vi "Raycaster_Run.vi"   [LabVIEW 2020]
uses:
  Controls/Raycaster_PlayLoop.ctl
  Controls/Game_State.ctl
  Controls/Player_LocationInfo.ctl
  Controls/Player_LocationInfoAxis.ctl
  Controls/Map_Position.ctl
  Controls/Map_Objects.ctl
  Controls/Map_Object.ctl
  Controls/Raycaster_DrawState.ctl
  Globals/FGV_TileVisibleEnum.ctl
  Raycaster_SetupDDA.vi
  Raycaster_RunDDA.vi
  Raycaster_DrawColumnSimple.vi
  Raycaster_CalcWallDistance.vi
  Raycaster_CalcWallHeight.vi
  Raycaster_GetSubBufferAddress.vi
  Raycaster_WriteFramebuffer.vi
  Globals/WIDTH.vi
  Math_Multiply_FXP.vi
  Math_Add_FXP.vi
  Math_Reciprocal.vi
  Math_Subtract_FXP.vi
  Globals/MAP_DIM.vi
  Map_ReadValue.vi
  Math_Divide_FXP.vi
  Globals/HEIGHT_DIV_2.vi
  Map_GetMaps.vi
  <vilib>/Utility/file.llb/Application Directory.vi
  <vilib>/eio/EIONode/EIONode.xnode
  <vilib>/rvi/DataTransferAndStorage/Container/XNode/niFpgaContainer.xnode
  <vilib>/rvi/Memory/Memory_Emulation/nirvimemoryEmulation.vi
  <vilib>/rvi/Memory/Memory_Emulation/nirvimemoryFastEmulation.vi
  <vilib>/rvi/eio/common/nirviEmuTemplateMethod_errors.vi
types:
  T1 = typedef "Map_Object.ctl" = cluster{"Distance":fxp<+/-,32,16>, "ID":u8, "Position":T2, "Visible":bool}
  T2 = typedef "Map_Position.ctl" = cluster{"X":fxp<+/-,32,16>, "Y":fxp<+/-,32,16>}
  T3 = typedef "Map_Objects.ctl" = cluster{"Objects":T1[], "Num Objects":i16, "Visible Objects":i16}
  T4 = typedef "Game_State.ctl" = cluster{"Map":u8, "Map Address":u32, "Location Info":T5, "Elevator":T2}
  T5 = typedef "Player_LocationInfo.ctl" = cluster{"X":T6, "Y":T6}
  T6 = typedef "Player_LocationInfoAxis.ctl" = cluster{"Position":fxp<+/-,32,16>, "Direction":fxp<+/-,32,16>, "Plane":fxp<+/-,32,16>}
  T7 = typedef "Raycaster_PlayLoop.ctl" = enum16{"Init", "Read Inputs", "Move Doors", "Move Walls", "Draw Walls", "Init Ray Caster", "Draw Scaled", "Draw Fizzle", "Update Screen"}
  T8 = typedef "Raycaster_DrawState.ctl" = cluster{"Buffer 0":u8[], "Buffer 1":u8[], "Buffer 2":u8[], "Buffer 3":u8[], "Wall Height 0":i16[], "Wall Height 1":i16[], "Wall Height 2":i16[], "Wall Height 3":i16[]}
  T9 = typedef "FGV_TileVisibleEnum.ctl" = enum16{"Reset", "Set Value", "Read Value"}
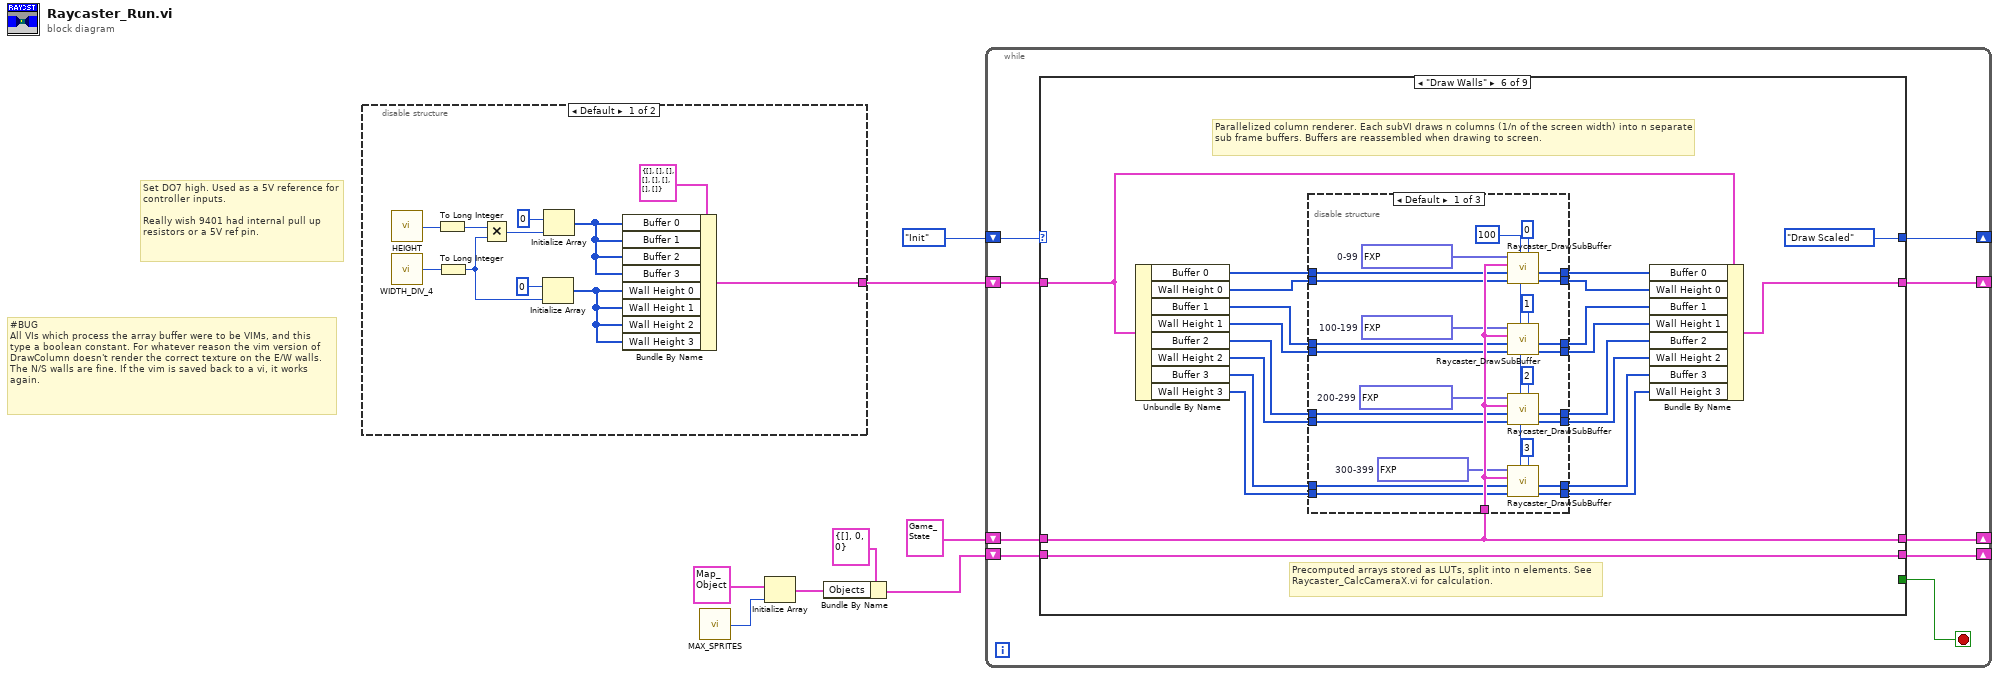
[diagram p0: block diagram]
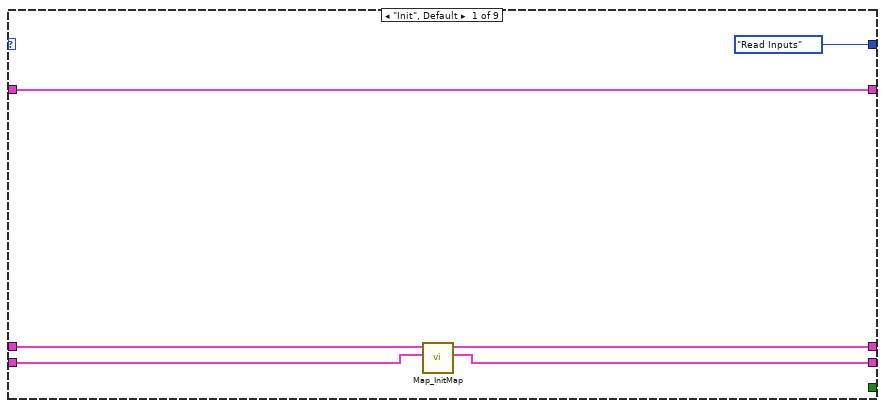
[diagram p2: hidden frame]
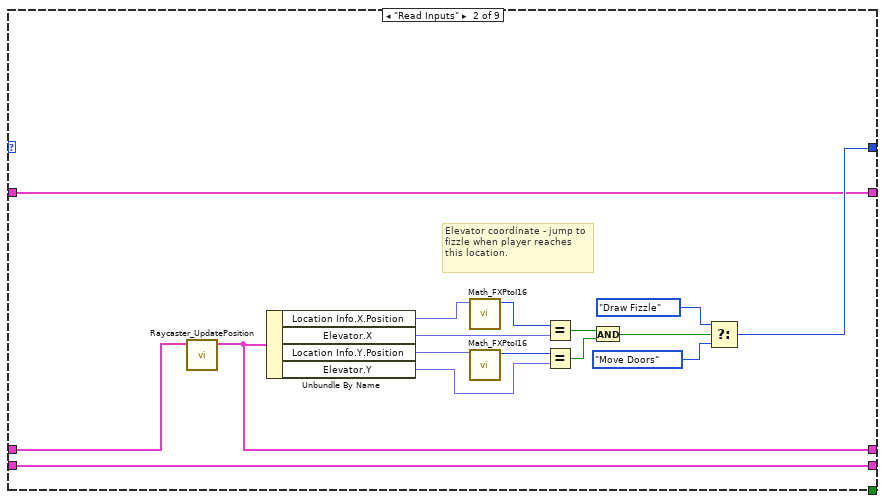
[diagram p3: hidden frame]
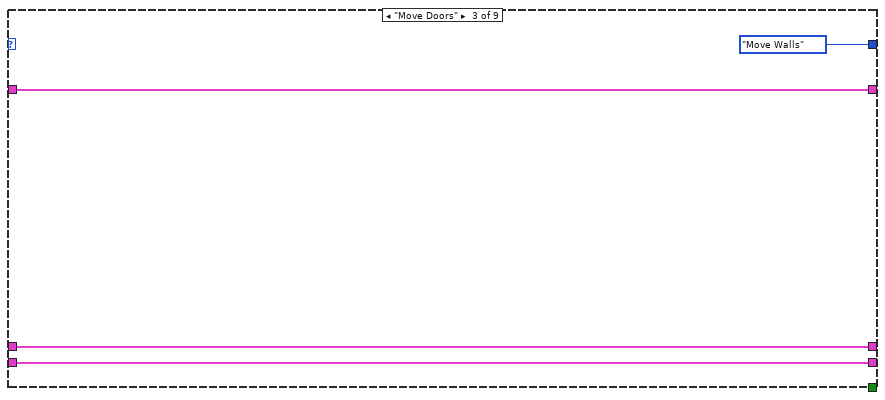
[diagram p4: hidden frame]
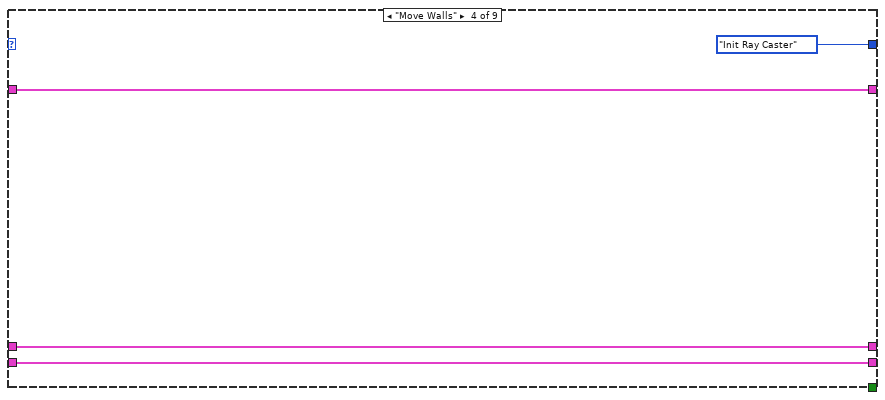
[diagram p5: hidden frame]
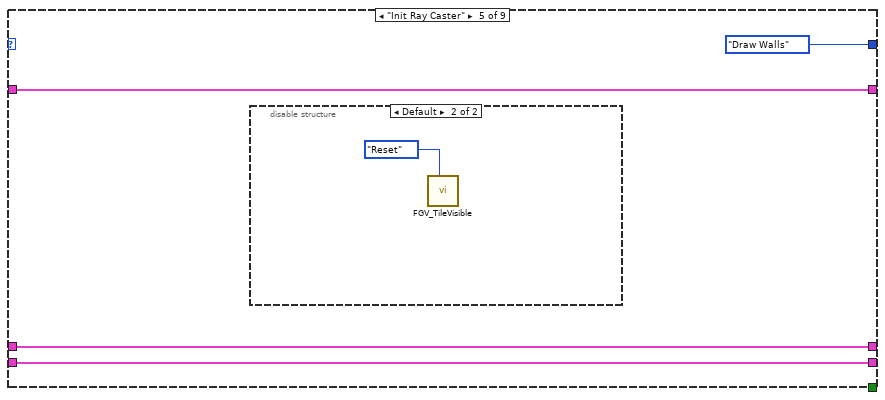
[diagram p6: hidden frame]
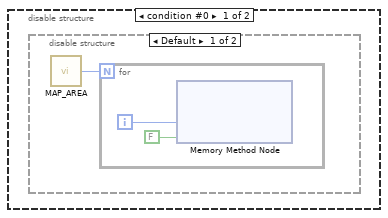
[diagram p7: hidden frame]
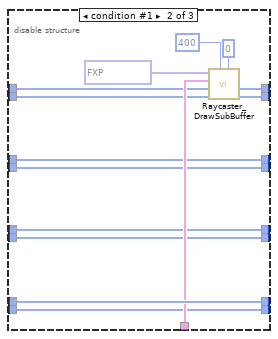
[diagram p9: hidden frame]
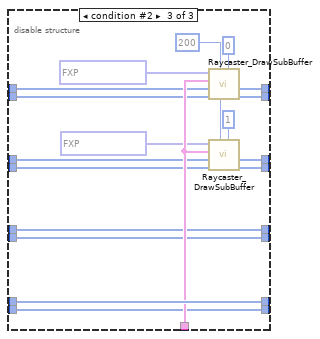
[diagram p10: hidden frame]
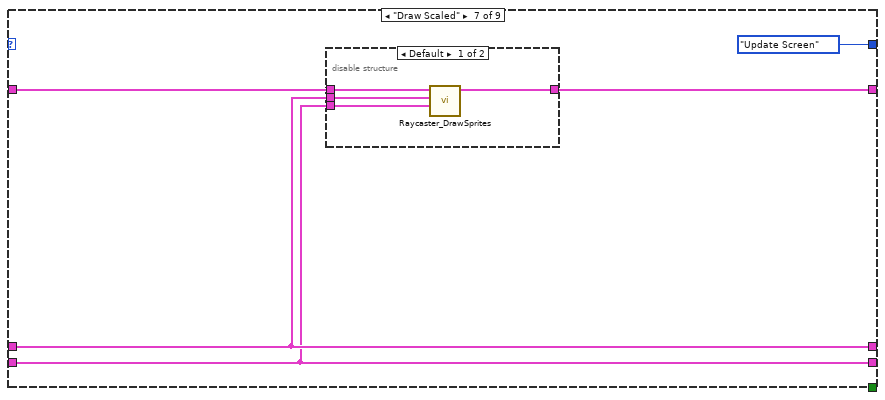
[diagram p11: hidden frame]
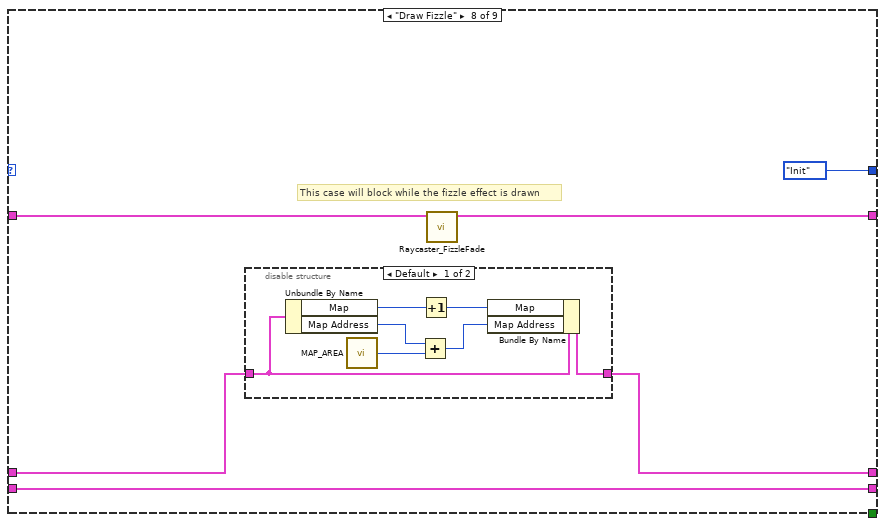
[diagram p13: hidden frame]
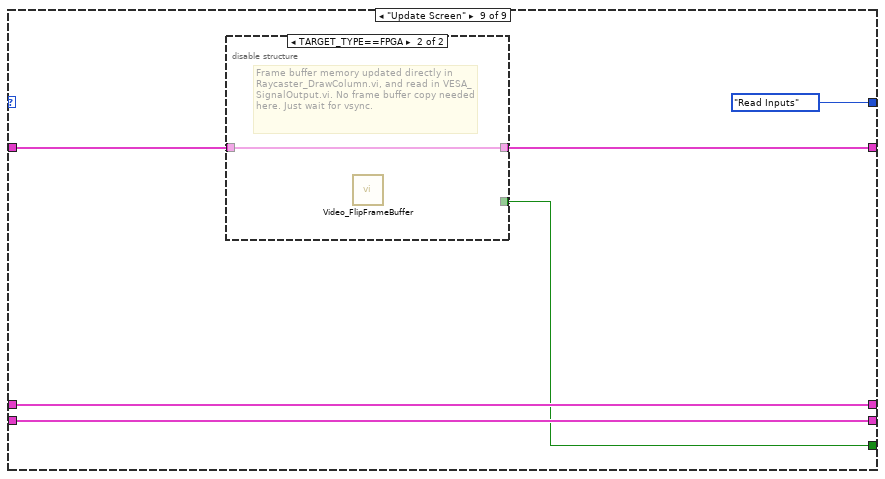
[diagram p15: hidden frame]
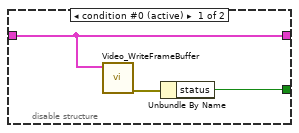
[diagram p16: hidden frame]
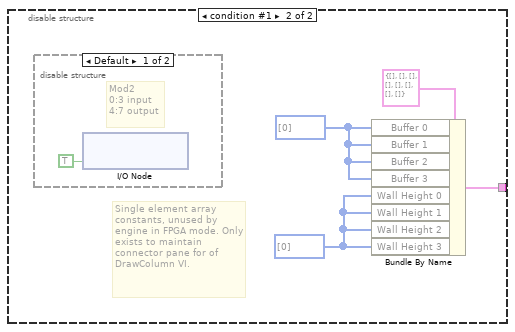
[diagram p17: hidden frame]
diagram:
  # "Set DO7 high. Used as a 5V reference for controller inputs.\n\nReally wish 9401 had internal pull up resistors or a 5V ref pin."
  # "#BUG\nAll VIs which process the array buffer were to be VIMs, and this type a boolean constant. For whatever reason the vim version of DrawColumn doesn't render the correct texture on the E/W walls. The N/S walls are fine. If the vim is saved back to a vi, it works again."
  n1 = disable-structure "Conditional Disable Structure" shown="Default" {
    disable-tunnel: [w15 w21] -> w2
    frame condition #0 (active) {
      n2 = call "HEIGHT.vi"() -> ("HEIGHT"=w19:i16)
      n3 = call "WIDTH_DIV_4.vi"() -> ("WIDTH_DIV_4"=w12:i16)
      n4 = To Long Integer(number=w19) -> (32bit integer=w18:i32)
      n5 = To Long Integer(number=w12) -> (32bit integer=w9:i32)
      n6 = Multiply(x=w18, y=w9) -> (x*y=w14:i32)
      n7 = Initialize Array(i16 0, w9) -> (w10:i16[])
      n8 = Initialize Array(u8 0, w14) -> (w13:u8[])
      n9 = Bundle By Name(cluster=T8 {"Buffer 0"=[], "Buffer 1"=[], "Buffer 2"=[], "Buffer 3"=[], "Wall Height 0"=[], "Wall Height 1"=[], "Wall Height 2"=[], "Wall Height 3"=[]} ("Frame buffers"), "Buffer 0"=w13, "Buffer 1"=w13, "Buffer 2"=w13, "Buffer 3"=w13, "Wall Height 0"=w10, "Wall Height 1"=w10, "Wall Height 2"=w10, "Wall Height 3"=w10) -> (w15:T8)
    }
    frame condition #1 {
      w20 = i16[] [0]
      w22 = u8[] [0]
      # "Single element array constants, unused by engine in FPGA mode. Only exists to maintain connector pane for of DrawColumn VI."
      n10 = disable-structure "Conditional Disable Structure" shown="Default" {
        frame condition #0 (active) {
          # "Mod2\n0:3 input\n4:7 output"
          n11 = xnode ("I/O Node")("Mod2/DIO7"=TRUE) -> ()  [unwired: 1 in, 1 out]
        }
        frame condition #1 {
        }
      }
      n12 = Bundle By Name(cluster=T8 {"Buffer 0"=[], "Buffer 1"=[], "Buffer 2"=[], "Buffer 3"=[], "Wall Height 0"=[], "Wall Height 1"=[], "Wall Height 2"=[], "Wall Height 3"=[]} ("Frame buffers"), "Buffer 0"=w22, "Buffer 1"=w22, "Buffer 2"=w22, "Buffer 3"=w22, "Wall Height 0"=w20, "Wall Height 1"=w20, "Wall Height 2"=w20, "Wall Height 3"=w20) -> (w21:T8)
    }
  }
  n13 = call "MAX_SPRITES.vi"() -> ("MAX_SPRITES"=w1:u8)
  n14 = Initialize Array(T1 {"Distance"=0.0, "ID"=0, "Position"={"X"=0.0, "Y"=0.0}, "Visible"=FALSE} ("Object"), w1) -> (w5:T1[])
  n15 = Bundle By Name(cluster=T3 {"Objects"=[], "Num Objects"=0, "Visible Objects"=0} ("Map Objects"), "Objects"=w5) -> (w3:T3)
  n16 = while {
    shift-right: [w29] -> _
    shift-left: T4 {"Map"=0, "Map Address"=0, "Location Info"={"X"={"Position"=0.0, "Direction"=0.0, "Plane"=0.0}, "Y"={"Position"=0.0, "Direction"=0.0, "Plane"=0.0}}, "Elevator"={"X"=0.0, "Y"=0.0}} ("Game State") -> [w30]
    shift-right: [w31] -> _
    shift-left: Raycaster_PlayLoop."Init" -> [w32]
    shift-right: [w26] -> _
    shift-left: w2 -> [w33]
    shift-right: [w27] -> _
    shift-left: w3 -> [w28]
    stop <- w25 stop-if-true
    n17 = case shown="\"Draw Walls\"" w32 {
      tunnel: w33 -> [w34 w51 w56 w60 w64 w89 w154 w162 w179]
      tunnel: [w37 w54 w58 w62 w66 w91 w153 w165 w180] -> w29
      tunnel: [Raycaster_PlayLoop."Read Inputs" w53 Raycaster_PlayLoop."Move Walls" Raycaster_PlayLoop."Init Ray Caster" Raycaster_PlayLoop."Draw Walls" Raycaster_PlayLoop."Draw Scaled" Raycaster_PlayLoop."Update Screen" Raycaster_PlayLoop."Init" Raycaster_PlayLoop."Read Inputs"] -> w31
      tunnel: w30 -> [w38 w55 w58 w62 w66 w91 w153 w164 w180]
      tunnel: w28 -> [w36 w52 w57 w61 w65 w90 w152 w163 w177]
      tunnel: [w35 w52 w57 w61 w65 w90 w152 w163 w177] -> w27
      tunnel: [w34 w51 w56 w60 w64 w88 w151 w161 w176] -> w26
      tunnel: [_ _ _ _ _ _ _ _ w175] -> w25
      frame "Init", Default {
        n18 = call "Map_InitMap.vi"("Map Objects In"=w36, "Game State In"=w38) -> ("Map Objects Out"=w35:T3, "Game State Out"=w37:T4)  [unwired: 8 in]
      }
      frame "Read Inputs" {
        # "Elevator coordinate - jump to fizzle when player reaches this location."
        n19 = call "Raycaster_UpdatePosition.vi"("Game State In"=w55) -> ("Game State Out"=w54:T4)  [unwired: 10 in]
        n20 = Unbundle By Name(w54) -> ("Location Info.X.Position"=w50:fxp<+/-,32,16>, "Elevator.X"=w41:fxp<+/-,32,16>, "Location Info.Y.Position"=w42:fxp<+/-,32,16>, "Elevator.Y"=w40:fxp<+/-,32,16>)
        n21 = call "Math_FXPtoI16.vi"("FXP"=w50) -> ("I16"=w49:i16)  [unwired: 10 in]
        n22 = call "Math_FXPtoI16.vi"("FXP"=w42) -> ("I16"=w48:i16)  [unwired: 10 in]
        n23 = Equal?(x=w49, y=w41) -> (x = y?=w47:bool)
        n24 = Equal?(x=w48, y=w40) -> (x = y?=w46:bool)
        n25 = And(x=w47, y=w46) -> (x .and. y?=w45:bool)
        n26 = Select(t=Raycaster_PlayLoop."Draw Fizzle", s=w45, f=Raycaster_PlayLoop."Move Doors") -> (s? t:f=w53:T7)
      }
      frame "Move Doors" {
      }
      frame "Move Walls" {
      }
      frame "Init Ray Caster" {
        n27 = disable-structure "Conditional Disable Structure" shown="Default" {
          frame condition #0 {
            n28 = disable-structure shown="Default" {
              frame condition #0 (active) {
                n29 = call "MAP_AREA.vi"() -> ("MAP_DIM"=w68:i16)
                n30 = for {
                  N: w68 -> [_]
                  i -> [w69]
                  n31 = xnode ("Memory Method Node")("Address"=w69, "Data"=FALSE) -> ()  [unwired: 1 in, 1 out]
                }
              }
              frame condition #1 {
              }
            }
          }
          frame condition #1 (active) {
            n32 = call "FGV_TileVisible.vi"("Tile Visible FGV"=FGV_TileVisibleEnum."Reset") -> ()  [unwired: 10 in, 1 out]
          }
        }
      }
      frame "Draw Walls" {
        # "Parallelized column renderer. Each subVI draws n columns (1/n of the screen width) into n separate sub frame buffers. Buffers are reassembled when drawing to screen."
        # "Precomputed arrays stored as LUTs, split into n elements. See Raycaster_CalcCameraX.vi for calculation."
        n33 = Unbundle By Name(w89) -> ("Buffer 0"=w87:u8[], "Wall Height 0"=w73:i16[], "Buffer 1"=w86:u8[], "Wall Height 1"=w75:i16[], "Buffer 2"=w83:u8[], "Wall Height 2"=w77:i16[], "Buffer 3"=w82:u8[], "Wall Height 3"=w79:i16[])
        n34 = disable-structure "Conditional Disable Structure" shown="Default" {
          disable-tunnel: w91 -> [w118 w130 w148]
          disable-tunnel: w87 -> [w117 w122 w144]
          disable-tunnel: w86 -> [w116 w128 w138]
          disable-tunnel: w83 -> [w115 w129 w147]
          disable-tunnel: w82 -> [w114 w131 w149]
          disable-tunnel: [w113 w121 w142] -> w85
          disable-tunnel: [w112 w128 w137] -> w84
          disable-tunnel: [w111 w129 w147] -> w81
          disable-tunnel: [w110 w131 w149] -> w80
          disable-tunnel: w79 -> [w104 w124 w133]
          disable-tunnel: [w103 w124 w133] -> w78
          disable-tunnel: w77 -> [w100 w125 w134]
          disable-tunnel: [w99 w125 w134] -> w76
          disable-tunnel: w75 -> [w97 w126 w135]
          disable-tunnel: [w96 w126 w136] -> w74
          disable-tunnel: w73 -> [w94 w120 w141]
          disable-tunnel: [w93 w119 w140] -> w72
          frame condition #0 (active) {
            w107 = i16 100 ("Column Offset")
            w105 = fxp<+/-,32,16>[] [0.5, 0.5049896240234375, 0.5099945068359375, 0.5149993896484375, 0.519989013671875, 0.524993896484375, 0.529998779296875, 0.5349884033203125, 0.5399932861328125, 0.5449981689453125, 0.54998779296875, 0.55499267578125, 0.55999755859375, 0.5649871826171875, 0.5699920654296875, 0.5749969482421875, 0.579986572265625, 0.584991455078125, 0.589996337890625, 0.5949859619140625, 0.5999908447265625, 0.6049957275390625, 0.6099853515625, 0.614990234375, 0.6199951171875, 0.625, 0.6299896240234375, 0.6349945068359375, 0.6399993896484375, 0.644989013671875, 0.649993896484375, 0.654998779296875, 0.6599884033203125, 0.6649932861328125, 0.6699981689453125, 0.67498779296875, 0.67999267578125, 0.68499755859375, 0.6899871826171875, 0.6949920654296875, 0.6999969482421875, 0.704986572265625, 0.709991455078125, 0.714996337890625, 0.7199859619140625, 0.7249908447265625, 0.7299957275390625, 0.7349853515625, 0.739990234375, 0.7449951171875, 0.75, 0.7549896240234375, 0.7599945068359375, 0.7649993896484375, 0.769989013671875, 0.774993896484375, 0.779998779296875, 0.7849884033203125, 0.7899932861328125, 0.7949981689453125, 0.79998779296875, 0.80499267578125, 0.80999755859375, 0.8149871826171875, 0.8199920654296875, 0.8249969482421875, 0.829986572265625, 0.834991455078125, 0.839996337890625, 0.8449859619140625, 0.8499908447265625, 0.8549957275390625, 0.8599853515625, 0.864990234375, 0.8699951171875, 0.875, 0.8799896240234375, 0.8849945068359375, 0.8899993896484375, 0.894989013671875, 0.899993896484375, 0.904998779296875, 0.9099884033203125, 0.9149932861328125, 0.9199981689453125, 0.92498779296875, 0.92999267578125, 0.93499755859375, 0.9399871826171875, 0.9449920654296875, 0.9499969482421875, 0.954986572265625, 0.959991455078125, 0.964996337890625, 0.9699859619140625, 0.9749908447265625, 0.9799957275390625, 0.9849853515625, 0.989990234375, 0.9949951171875]  # 300-399
            w106 = fxp<+/-,32,16>[] [0.0, 0.0049896240234375, 0.0099945068359375, 0.0149993896484375, 0.019989013671875, 0.024993896484375, 0.029998779296875, 0.0349884033203125, 0.0399932861328125, 0.0449981689453125, 0.04998779296875, 0.05499267578125, 0.05999755859375, 0.0649871826171875, 0.0699920654296875, 0.0749969482421875, 0.079986572265625, 0.084991455078125, 0.089996337890625, 0.0949859619140625, 0.0999908447265625, 0.1049957275390625, 0.1099853515625, 0.114990234375, 0.1199951171875, 0.125, 0.1299896240234375, 0.1349945068359375, 0.1399993896484375, 0.144989013671875, 0.149993896484375, 0.154998779296875, 0.1599884033203125, 0.1649932861328125, 0.1699981689453125, 0.17498779296875, 0.17999267578125, 0.18499755859375, 0.1899871826171875, 0.1949920654296875, 0.1999969482421875, 0.204986572265625, 0.209991455078125, 0.214996337890625, 0.2199859619140625, 0.2249908447265625, 0.2299957275390625, 0.2349853515625, 0.239990234375, 0.2449951171875, 0.25, 0.2549896240234375, 0.2599945068359375, 0.2649993896484375, 0.269989013671875, 0.274993896484375, 0.279998779296875, 0.2849884033203125, 0.2899932861328125, 0.2949981689453125, 0.29998779296875, 0.30499267578125, 0.30999755859375, 0.3149871826171875, 0.3199920654296875, 0.3249969482421875, 0.329986572265625, 0.334991455078125, 0.339996337890625, 0.3449859619140625, 0.3499908447265625, 0.3549957275390625, 0.3599853515625, 0.364990234375, 0.3699951171875, 0.375, 0.3799896240234375, 0.3849945068359375, 0.3899993896484375, 0.394989013671875, 0.399993896484375, 0.404998779296875, 0.4099884033203125, 0.4149932861328125, 0.4199981689453125, 0.42498779296875, 0.42999267578125, 0.43499755859375, 0.4399871826171875, 0.4449920654296875, 0.4499969482421875, 0.454986572265625, 0.459991455078125, 0.464996337890625, 0.4699859619140625, 0.4749908447265625, 0.4799957275390625, 0.4849853515625, 0.489990234375, 0.4949951171875]  # 200-299
            w108 = fxp<+/-,32,16>[] [-0.5, -0.4950103759765625, -0.4900054931640625, -0.4850006103515625, -0.480010986328125, -0.475006103515625, -0.470001220703125, -0.4650115966796875, -0.4600067138671875, -0.4550018310546875, -0.45001220703125, -0.44500732421875, -0.44000244140625, -0.4350128173828125, -0.4300079345703125, -0.4250030517578125, -0.420013427734375, -0.415008544921875, -0.410003662109375, -0.4050140380859375, -0.4000091552734375, -0.3950042724609375, -0.3900146484375, -0.385009765625, -0.3800048828125, -0.375, -0.3700103759765625, -0.3650054931640625, -0.3600006103515625, -0.355010986328125, -0.350006103515625, -0.345001220703125, -0.3400115966796875, -0.3350067138671875, -0.3300018310546875, -0.32501220703125, -0.32000732421875, -0.31500244140625, -0.3100128173828125, -0.3050079345703125, -0.3000030517578125, -0.295013427734375, -0.290008544921875, -0.285003662109375, -0.2800140380859375, -0.2750091552734375, -0.2700042724609375, -0.2650146484375, -0.260009765625, -0.2550048828125, -0.25, -0.2450103759765625, -0.2400054931640625, -0.2350006103515625, -0.230010986328125, -0.225006103515625, -0.220001220703125, -0.2150115966796875, -0.2100067138671875, -0.2050018310546875, -0.20001220703125, -0.19500732421875, -0.19000244140625, -0.1850128173828125, -0.1800079345703125, -0.1750030517578125, -0.170013427734375, -0.165008544921875, -0.160003662109375, -0.1550140380859375, -0.1500091552734375, -0.1450042724609375, -0.1400146484375, -0.135009765625, -0.1300048828125, -0.125, -0.1200103759765625, -0.1150054931640625, -0.1100006103515625, -0.105010986328125, -0.100006103515625, -0.095001220703125, -0.0900115966796875, -0.0850067138671875, -0.0800018310546875, -0.07501220703125, -0.07000732421875, -0.06500244140625, -0.0600128173828125, -0.0550079345703125, -0.0500030517578125, -0.045013427734375, -0.040008544921875, -0.035003662109375, -0.0300140380859375, -0.0250091552734375, -0.0200042724609375, -0.0150146484375, -0.010009765625, -0.0050048828125]  # 100-199
            w109 = fxp<+/-,32,16>[] [-1.0, -0.9950103759765625, -0.9900054931640625, -0.9850006103515625, -0.980010986328125, -0.975006103515625, -0.970001220703125, -0.9650115966796875, -0.9600067138671875, -0.9550018310546875, -0.95001220703125, -0.94500732421875, -0.94000244140625, -0.9350128173828125, -0.9300079345703125, -0.9250030517578125, -0.920013427734375, -0.915008544921875, -0.910003662109375, -0.9050140380859375, -0.9000091552734375, -0.8950042724609375, -0.8900146484375, -0.885009765625, -0.8800048828125, -0.875, -0.8700103759765625, -0.8650054931640625, -0.8600006103515625, -0.855010986328125, -0.850006103515625, -0.845001220703125, -0.8400115966796875, -0.8350067138671875, -0.8300018310546875, -0.82501220703125, -0.82000732421875, -0.81500244140625, -0.8100128173828125, -0.8050079345703125, -0.8000030517578125, -0.795013427734375, -0.790008544921875, -0.785003662109375, -0.7800140380859375, -0.7750091552734375, -0.7700042724609375, -0.7650146484375, -0.760009765625, -0.7550048828125, -0.75, -0.7450103759765625, -0.7400054931640625, -0.7350006103515625, -0.730010986328125, -0.725006103515625, -0.720001220703125, -0.7150115966796875, -0.7100067138671875, -0.7050018310546875, -0.70001220703125, -0.69500732421875, -0.69000244140625, -0.6850128173828125, -0.6800079345703125, -0.6750030517578125, -0.670013427734375, -0.665008544921875, -0.660003662109375, -0.6550140380859375, -0.6500091552734375, -0.6450042724609375, -0.6400146484375, -0.635009765625, -0.6300048828125, -0.625, -0.6200103759765625, -0.6150054931640625, -0.6100006103515625, -0.605010986328125, -0.600006103515625, -0.595001220703125, -0.5900115966796875, -0.5850067138671875, -0.5800018310546875, -0.57501220703125, -0.57000732421875, -0.56500244140625, -0.5600128173828125, -0.5550079345703125, -0.5500030517578125, -0.545013427734375, -0.540008544921875, -0.535003662109375, -0.5300140380859375, -0.5250091552734375, -0.5200042724609375, -0.5150146484375, -0.510009765625, -0.5050048828125]  # 0-99
            n35 = call "Raycaster_DrawSubBuffer.vi"("Sub Buffer"=u8 0, "Num Columns"=w107, "Wall Height In"=w94, "Buffer In"=w117, "Game State"=w118, "Camera X"=w109) -> ("Wall Height Out"=w93:i16[], "Buffer Out"=w113:u8[])  [unwired: 4 in]
            n36 = call "Raycaster_DrawSubBuffer.vi"("Sub Buffer"=u8 1 ("Column Offset"), "Num Columns"=w107, "Wall Height In"=w97, "Buffer In"=w116, "Game State"=w118, "Camera X"=w108) -> ("Wall Height Out"=w96:i16[], "Buffer Out"=w112:u8[])  [unwired: 4 in]
            n37 = call "Raycaster_DrawSubBuffer.vi"("Sub Buffer"=u8 2 ("Column Offset"), "Num Columns"=w107, "Wall Height In"=w100, "Buffer In"=w115, "Game State"=w118, "Camera X"=w106) -> ("Wall Height Out"=w99:i16[], "Buffer Out"=w111:u8[])  [unwired: 4 in]
            n38 = call "Raycaster_DrawSubBuffer.vi"("Sub Buffer"=u8 3 ("Column Offset"), "Num Columns"=w107, "Wall Height In"=w104, "Buffer In"=w114, "Game State"=w118, "Camera X"=w105) -> ("Wall Height Out"=w103:i16[], "Buffer Out"=w110:u8[])  [unwired: 4 in]
          }
          frame condition #1 {
            n39 = call "Raycaster_DrawSubBuffer.vi"("Sub Buffer"=u8 0, "Num Columns"=i16 400 ("Column Offset"), "Wall Height In"=w120, "Buffer In"=w122, "Game State"=w130, "Camera X"=fxp<+/-,32,16>[] [-1.0, -0.9950103759765625, -0.9900054931640625, -0.9850006103515625, -0.980010986328125, -0.975006103515625, -0.970001220703125, -0.9650115966796875, -0.9600067138671875, -0.9550018310546875, -0.95001220703125, -0.94500732421875, -0.94000244140625, -0.9350128173828125, -0.9300079345703125, -0.9250030517578125, -0.920013427734375, -0.915008544921875, -0.910003662109375, -0.9050140380859375, -0.9000091552734375, -0.8950042724609375, -0.8900146484375, -0.885009765625, -0.8800048828125, -0.875, -0.8700103759765625, -0.8650054931640625, -0.8600006103515625, -0.855010986328125, -0.850006103515625, -0.845001220703125, -0.8400115966796875, -0.8350067138671875, -0.8300018310546875, -0.82501220703125, -0.82000732421875, -0.81500244140625, -0.8100128173828125, -0.8050079345703125, -0.8000030517578125, -0.795013427734375, -0.790008544921875, -0.785003662109375, -0.7800140380859375, -0.7750091552734375, -0.7700042724609375, -0.7650146484375, -0.760009765625, -0.7550048828125, -0.75, -0.7450103759765625, -0.7400054931640625, -0.7350006103515625, -0.730010986328125, -0.725006103515625, -0.720001220703125, -0.7150115966796875, -0.7100067138671875, -0.7050018310546875, -0.70001220703125, -0.69500732421875, -0.69000244140625, -0.6850128173828125, -0.6800079345703125, -0.6750030517578125, -0.670013427734375, -0.665008544921875, -0.660003662109375, -0.6550140380859375, -0.6500091552734375, -0.6450042724609375, -0.6400146484375, -0.635009765625, -0.6300048828125, -0.625, -0.6200103759765625, -0.6150054931640625, -0.6100006103515625, -0.605010986328125, -0.600006103515625, -0.595001220703125, -0.5900115966796875, -0.5850067138671875, -0.5800018310546875, -0.57501220703125, -0.57000732421875, -0.56500244140625, -0.5600128173828125, -0.5550079345703125, -0.5500030517578125, -0.545013427734375, -0.540008544921875, -0.535003662109375, -0.5300140380859375, -0.5250091552734375, -0.5200042724609375, -0.5150146484375, -0.510009765625, -0.5050048828125, -0.5, -0.4950103759765625, -0.4900054931640625, -0.4850006103515625, -0.480010986328125, -0.475006103515625, -0.470001220703125, -0.4650115966796875, -0.4600067138671875, -0.4550018310546875, -0.45001220703125, -0.44500732421875, -0.44000244140625, -0.4350128173828125, -0.4300079345703125, -0.4250030517578125, -0.420013427734375, -0.415008544921875, -0.410003662109375, -0.4050140380859375, -0.4000091552734375, -0.3950042724609375, -0.3900146484375, -0.385009765625, -0.3800048828125, -0.375, -0.3700103759765625, -0.3650054931640625, -0.3600006103515625, -0.355010986328125, -0.350006103515625, -0.345001220703125, -0.3400115966796875, -0.3350067138671875, -0.3300018310546875, -0.32501220703125, -0.32000732421875, -0.31500244140625, -0.3100128173828125, -0.3050079345703125, -0.3000030517578125, -0.295013427734375, -0.290008544921875, -0.285003662109375, -0.2800140380859375, -0.2750091552734375, -0.2700042724609375, -0.2650146484375, -0.260009765625, -0.2550048828125, -0.25, -0.2450103759765625, -0.2400054931640625, -0.2350006103515625, -0.230010986328125, -0.225006103515625, -0.220001220703125, -0.2150115966796875, -0.2100067138671875, -0.2050018310546875, -0.20001220703125, -0.19500732421875, -0.19000244140625, -0.1850128173828125, -0.1800079345703125, -0.1750030517578125, -0.170013427734375, -0.165008544921875, -0.160003662109375, -0.1550140380859375, -0.1500091552734375, -0.1450042724609375, -0.1400146484375, -0.135009765625, -0.1300048828125, -0.125, -0.1200103759765625, -0.1150054931640625, -0.1100006103515625, -0.105010986328125, -0.100006103515625, -0.095001220703125, -0.0900115966796875, -0.0850067138671875, -0.0800018310546875, -0.07501220703125, -0.07000732421875, -0.06500244140625, -0.0600128173828125, -0.0550079345703125, -0.0500030517578125, -0.045013427734375, -0.040008544921875, -0.035003662109375, -0.0300140380859375, -0.0250091552734375, -0.0200042724609375, -0.0150146484375, -0.010009765625, -0.0050048828125, 0.0, 0.0049896240234375, 0.0099945068359375, 0.0149993896484375, 0.019989013671875, 0.024993896484375, 0.029998779296875, 0.0349884033203125, 0.0399932861328125, 0.0449981689453125, 0.04998779296875, 0.05499267578125, 0.05999755859375, 0.0649871826171875, 0.0699920654296875, 0.0749969482421875, 0.079986572265625, 0.084991455078125, 0.089996337890625, 0.0949859619140625, 0.0999908447265625, 0.1049957275390625, 0.1099853515625, 0.114990234375, 0.1199951171875, 0.125, 0.1299896240234375, 0.1349945068359375, 0.1399993896484375, 0.144989013671875, 0.149993896484375, 0.154998779296875, 0.1599884033203125, 0.1649932861328125, 0.1699981689453125, 0.17498779296875, 0.17999267578125, 0.18499755859375, 0.1899871826171875, 0.1949920654296875, 0.1999969482421875, 0.204986572265625, 0.209991455078125, 0.214996337890625, 0.2199859619140625, 0.2249908447265625, 0.2299957275390625, 0.2349853515625, 0.239990234375, 0.2449951171875, 0.25, 0.2549896240234375, 0.2599945068359375, 0.2649993896484375, 0.269989013671875, 0.274993896484375, 0.279998779296875, 0.2849884033203125, 0.2899932861328125, 0.2949981689453125, 0.29998779296875, 0.30499267578125, 0.30999755859375, 0.3149871826171875, 0.3199920654296875, 0.3249969482421875, 0.329986572265625, 0.334991455078125, 0.339996337890625, 0.3449859619140625, 0.3499908447265625, 0.3549957275390625, 0.3599853515625, 0.364990234375, 0.3699951171875, 0.375, 0.3799896240234375, 0.3849945068359375, 0.3899993896484375, 0.394989013671875, 0.399993896484375, 0.404998779296875, 0.4099884033203125, 0.4149932861328125, 0.4199981689453125, 0.42498779296875, 0.42999267578125, 0.43499755859375, 0.4399871826171875, 0.4449920654296875, 0.4499969482421875, 0.454986572265625, 0.459991455078125, 0.464996337890625, 0.4699859619140625, 0.4749908447265625, 0.4799957275390625, 0.4849853515625, 0.489990234375, 0.4949951171875, 0.5, 0.5049896240234375, 0.5099945068359375, 0.5149993896484375, 0.519989013671875, 0.524993896484375, 0.529998779296875, 0.5349884033203125, 0.5399932861328125, 0.5449981689453125, 0.54998779296875, 0.55499267578125, 0.55999755859375, 0.5649871826171875, 0.5699920654296875, 0.5749969482421875, 0.579986572265625, 0.584991455078125, 0.589996337890625, 0.5949859619140625, 0.5999908447265625, 0.6049957275390625, 0.6099853515625, 0.614990234375, 0.6199951171875, 0.625, 0.6299896240234375, 0.6349945068359375, 0.6399993896484375, 0.644989013671875, 0.649993896484375, 0.654998779296875, 0.6599884033203125, 0.6649932861328125, 0.6699981689453125, 0.67498779296875, 0.67999267578125, 0.68499755859375, 0.6899871826171875, 0.6949920654296875, 0.6999969482421875, 0.704986572265625, 0.709991455078125, 0.714996337890625, 0.7199859619140625, 0.7249908447265625, 0.7299957275390625, 0.7349853515625, 0.739990234375, 0.7449951171875, 0.75, 0.7549896240234375, 0.7599945068359375, 0.7649993896484375, 0.769989013671875, 0.774993896484375, 0.779998779296875, 0.7849884033203125, 0.7899932861328125, 0.7949981689453125, 0.79998779296875, 0.80499267578125, 0.80999755859375, 0.8149871826171875, 0.8199920654296875, 0.8249969482421875, 0.829986572265625, 0.834991455078125, 0.839996337890625, 0.8449859619140625, 0.8499908447265625, 0.8549957275390625, 0.8599853515625, 0.864990234375, 0.8699951171875, 0.875, 0.8799896240234375, 0.8849945068359375, 0.8899993896484375, 0.894989013671875, 0.899993896484375, 0.904998779296875, 0.9099884033203125, 0.9149932861328125, 0.9199981689453125, 0.92498779296875, 0.92999267578125, 0.93499755859375, 0.9399871826171875, 0.9449920654296875, 0.9499969482421875, 0.954986572265625, 0.959991455078125, 0.964996337890625, 0.9699859619140625, 0.9749908447265625, 0.9799957275390625, 0.9849853515625, 0.989990234375, 0.9949951171875] ("appended array")) -> ("Wall Height Out"=w119:i16[], "Buffer Out"=w121:u8[])  [unwired: 4 in]
          }
          frame condition #2 {
            w150 = i16 200 ("Column Offset")
            n40 = call "Raycaster_DrawSubBuffer.vi"("Sub Buffer"=u8 0 ("Column Offset"), "Num Columns"=w150, "Wall Height In"=w141, "Buffer In"=w144, "Game State"=w148, "Camera X"=fxp<+/-,32,16>[] [-1.0, -0.9950103759765625, -0.9900054931640625, -0.9850006103515625, -0.980010986328125, -0.975006103515625, -0.970001220703125, -0.9650115966796875, -0.9600067138671875, -0.9550018310546875, -0.95001220703125, -0.94500732421875, -0.94000244140625, -0.9350128173828125, -0.9300079345703125, -0.9250030517578125, -0.920013427734375, -0.915008544921875, -0.910003662109375, -0.9050140380859375, -0.9000091552734375, -0.8950042724609375, -0.8900146484375, -0.885009765625, -0.8800048828125, -0.875, -0.8700103759765625, -0.8650054931640625, -0.8600006103515625, -0.855010986328125, -0.850006103515625, -0.845001220703125, -0.8400115966796875, -0.8350067138671875, -0.8300018310546875, -0.82501220703125, -0.82000732421875, -0.81500244140625, -0.8100128173828125, -0.8050079345703125, -0.8000030517578125, -0.795013427734375, -0.790008544921875, -0.785003662109375, -0.7800140380859375, -0.7750091552734375, -0.7700042724609375, -0.7650146484375, -0.760009765625, -0.7550048828125, -0.75, -0.7450103759765625, -0.7400054931640625, -0.7350006103515625, -0.730010986328125, -0.725006103515625, -0.720001220703125, -0.7150115966796875, -0.7100067138671875, -0.7050018310546875, -0.70001220703125, -0.69500732421875, -0.69000244140625, -0.6850128173828125, -0.6800079345703125, -0.6750030517578125, -0.670013427734375, -0.665008544921875, -0.660003662109375, -0.6550140380859375, -0.6500091552734375, -0.6450042724609375, -0.6400146484375, -0.635009765625, -0.6300048828125, -0.625, -0.6200103759765625, -0.6150054931640625, -0.6100006103515625, -0.605010986328125, -0.600006103515625, -0.595001220703125, -0.5900115966796875, -0.5850067138671875, -0.5800018310546875, -0.57501220703125, -0.57000732421875, -0.56500244140625, -0.5600128173828125, -0.5550079345703125, -0.5500030517578125, -0.545013427734375, -0.540008544921875, -0.535003662109375, -0.5300140380859375, -0.5250091552734375, -0.5200042724609375, -0.5150146484375, -0.510009765625, -0.5050048828125, -0.5, -0.4950103759765625, -0.4900054931640625, -0.4850006103515625, -0.480010986328125, -0.475006103515625, -0.470001220703125, -0.4650115966796875, -0.4600067138671875, -0.4550018310546875, -0.45001220703125, -0.44500732421875, -0.44000244140625, -0.4350128173828125, -0.4300079345703125, -0.4250030517578125, -0.420013427734375, -0.415008544921875, -0.410003662109375, -0.4050140380859375, -0.4000091552734375, -0.3950042724609375, -0.3900146484375, -0.385009765625, -0.3800048828125, -0.375, -0.3700103759765625, -0.3650054931640625, -0.3600006103515625, -0.355010986328125, -0.350006103515625, -0.345001220703125, -0.3400115966796875, -0.3350067138671875, -0.3300018310546875, -0.32501220703125, -0.32000732421875, -0.31500244140625, -0.3100128173828125, -0.3050079345703125, -0.3000030517578125, -0.295013427734375, -0.290008544921875, -0.285003662109375, -0.2800140380859375, -0.2750091552734375, -0.2700042724609375, -0.2650146484375, -0.260009765625, -0.2550048828125, -0.25, -0.2450103759765625, -0.2400054931640625, -0.2350006103515625, -0.230010986328125, -0.225006103515625, -0.220001220703125, -0.2150115966796875, -0.2100067138671875, -0.2050018310546875, -0.20001220703125, -0.19500732421875, -0.19000244140625, -0.1850128173828125, -0.1800079345703125, -0.1750030517578125, -0.170013427734375, -0.165008544921875, -0.160003662109375, -0.1550140380859375, -0.1500091552734375, -0.1450042724609375, -0.1400146484375, -0.135009765625, -0.1300048828125, -0.125, -0.1200103759765625, -0.1150054931640625, -0.1100006103515625, -0.105010986328125, -0.100006103515625, -0.095001220703125, -0.0900115966796875, -0.0850067138671875, -0.0800018310546875, -0.07501220703125, -0.07000732421875, -0.06500244140625, -0.0600128173828125, -0.0550079345703125, -0.0500030517578125, -0.045013427734375, -0.040008544921875, -0.035003662109375, -0.0300140380859375, -0.0250091552734375, -0.0200042724609375, -0.0150146484375, -0.010009765625, -0.0050048828125] ("appended array 2")) -> ("Wall Height Out"=w140:i16[], "Buffer Out"=w142:u8[])  [unwired: 4 in]
            n41 = call "Raycaster_DrawSubBuffer.vi"("Sub Buffer"=u8 1, "Num Columns"=w150, "Wall Height In"=w135, "Buffer In"=w138, "Game State"=w148, "Camera X"=fxp<+/-,32,16>[] [0.0, 0.0049896240234375, 0.0099945068359375, 0.0149993896484375, 0.019989013671875, 0.024993896484375, 0.029998779296875, 0.0349884033203125, 0.0399932861328125, 0.0449981689453125, 0.04998779296875, 0.05499267578125, 0.05999755859375, 0.0649871826171875, 0.0699920654296875, 0.0749969482421875, 0.079986572265625, 0.084991455078125, 0.089996337890625, 0.0949859619140625, 0.0999908447265625, 0.1049957275390625, 0.1099853515625, 0.114990234375, 0.1199951171875, 0.125, 0.1299896240234375, 0.1349945068359375, 0.1399993896484375, 0.144989013671875, 0.149993896484375, 0.154998779296875, 0.1599884033203125, 0.1649932861328125, 0.1699981689453125, 0.17498779296875, 0.17999267578125, 0.18499755859375, 0.1899871826171875, 0.1949920654296875, 0.1999969482421875, 0.204986572265625, 0.209991455078125, 0.214996337890625, 0.2199859619140625, 0.2249908447265625, 0.2299957275390625, 0.2349853515625, 0.239990234375, 0.2449951171875, 0.25, 0.2549896240234375, 0.2599945068359375, 0.2649993896484375, 0.269989013671875, 0.274993896484375, 0.279998779296875, 0.2849884033203125, 0.2899932861328125, 0.2949981689453125, 0.29998779296875, 0.30499267578125, 0.30999755859375, 0.3149871826171875, 0.3199920654296875, 0.3249969482421875, 0.329986572265625, 0.334991455078125, 0.339996337890625, 0.3449859619140625, 0.3499908447265625, 0.3549957275390625, 0.3599853515625, 0.364990234375, 0.3699951171875, 0.375, 0.3799896240234375, 0.3849945068359375, 0.3899993896484375, 0.394989013671875, 0.399993896484375, 0.404998779296875, 0.4099884033203125, 0.4149932861328125, 0.4199981689453125, 0.42498779296875, 0.42999267578125, 0.43499755859375, 0.4399871826171875, 0.4449920654296875, 0.4499969482421875, 0.454986572265625, 0.459991455078125, 0.464996337890625, 0.4699859619140625, 0.4749908447265625, 0.4799957275390625, 0.4849853515625, 0.489990234375, 0.4949951171875, 0.5, 0.5049896240234375, 0.5099945068359375, 0.5149993896484375, 0.519989013671875, 0.524993896484375, 0.529998779296875, 0.5349884033203125, 0.5399932861328125, 0.5449981689453125, 0.54998779296875, 0.55499267578125, 0.55999755859375, 0.5649871826171875, 0.5699920654296875, 0.5749969482421875, 0.579986572265625, 0.584991455078125, 0.589996337890625, 0.5949859619140625, 0.5999908447265625, 0.6049957275390625, 0.6099853515625, 0.614990234375, 0.6199951171875, 0.625, 0.6299896240234375, 0.6349945068359375, 0.6399993896484375, 0.644989013671875, 0.649993896484375, 0.654998779296875, 0.6599884033203125, 0.6649932861328125, 0.6699981689453125, 0.67498779296875, 0.67999267578125, 0.68499755859375, 0.6899871826171875, 0.6949920654296875, 0.6999969482421875, 0.704986572265625, 0.709991455078125, 0.714996337890625, 0.7199859619140625, 0.7249908447265625, 0.7299957275390625, 0.7349853515625, 0.739990234375, 0.7449951171875, 0.75, 0.7549896240234375, 0.7599945068359375, 0.7649993896484375, 0.769989013671875, 0.774993896484375, 0.779998779296875, 0.7849884033203125, 0.7899932861328125, 0.7949981689453125, 0.79998779296875, 0.80499267578125, 0.80999755859375, 0.8149871826171875, 0.8199920654296875, 0.8249969482421875, 0.829986572265625, 0.834991455078125, 0.839996337890625, 0.8449859619140625, 0.8499908447265625, 0.8549957275390625, 0.8599853515625, 0.864990234375, 0.8699951171875, 0.875, 0.8799896240234375, 0.8849945068359375, 0.8899993896484375, 0.894989013671875, 0.899993896484375, 0.904998779296875, 0.9099884033203125, 0.9149932861328125, 0.9199981689453125, 0.92498779296875, 0.92999267578125, 0.93499755859375, 0.9399871826171875, 0.9449920654296875, 0.9499969482421875, 0.954986572265625, 0.959991455078125, 0.964996337890625, 0.9699859619140625, 0.9749908447265625, 0.9799957275390625, 0.9849853515625, 0.989990234375, 0.9949951171875] ("appended array")) -> ("Wall Height Out"=w136:i16[], "Buffer Out"=w137:u8[])  [unwired: 4 in]
          }
        }
        n42 = Bundle By Name(cluster=w89, "Buffer 0"=w85, "Wall Height 0"=w72, "Buffer 1"=w84, "Wall Height 1"=w74, "Buffer 2"=w81, "Wall Height 2"=w76, "Buffer 3"=w80, "Wall Height 3"=w78) -> (w88:T8)
      }
      frame "Draw Scaled" {
        n43 = disable-structure shown="Default" {
          disable-tunnel: w154 -> [w159 w160]
          disable-tunnel: w153 -> [w158 _]
          disable-tunnel: w152 -> [w157 _]
          disable-tunnel: [w156 w160] -> w151
          frame condition #0 (active) {
            n44 = call "Raycaster_DrawSprites.vi"("Decorations In"=w157, "Game State"=w158, "Frame Buffers In"=w159) -> ("Frame Buffers Out"=w156:T8)  [unwired: 8 in]
          }
          frame condition #1 {
          }
        }
      }
      frame "Draw Fizzle" {
        # "This case will block while the fizzle effect is drawn"
        n45 = disable-structure "Conditional Disable Structure" shown="Default" {
          disable-tunnel: [w173 w174] -> w165
          disable-tunnel: w164 -> [w172 w174]
          frame condition #0 (active) {
            n46 = Unbundle By Name(w172) -> ("Map"=w171:u8, "Map Address"=w169:u32)
            n47 = call "MAP_AREA.vi"() -> ("MAP_DIM"=w168:i16)
            n48 = Add(x=w169, y=w168) -> (x+y=w167:u32)
            n49 = Increment(x=w171) -> (x+1=w170:u8)
            n50 = Bundle By Name(cluster=w172, "Map"=w170, "Map Address"=w167) -> (w173:T4)
          }
          frame condition #1 {
            # "Only one map on FPGA.\n\n#TODO\nImlement RLE on maps, the same as sprites"
          }
        }
        n51 = call "Raycaster_FizzleFade.vi"("Frame Buffers In"=w162) -> ("Frame Buffers Out"=w161:T8)  [unwired: 10 in]
      }
      frame "Update Screen" {
        n52 = disable-structure "Conditional Disable Structure" shown="TARGET_TYPE==FPGA" {
          disable-tunnel: w179 -> [w183 w184]
          disable-tunnel: [w183 w184] -> w176
          disable-tunnel: [w181 _] -> w175
          frame condition #0 (active) {
            n53 = call "Video_WriteFrameBuffer.vi"("Frame Buffers"=w183) -> ("error out"=w182:errorcluster)  [unwired: 10 in]
            n54 = Unbundle By Name(w182) -> ("status"=w181:bool)
          }
          frame condition #1 {
            # "Frame buffer memory updated directly in Raycaster_DrawColumn.vi, and read in VESA_SignalOutput.vi. No frame buffer copy needed here. Just wait for vsync."
            n55 = call "Video_FlipFrameBuffer.vi"() -> ()  [unwired: 11 in, 1 out]
          }
        }
      }
    }
  }
